vi "Display Print Dialog.vi"(8 "error in (no error)":errorcluster, 10 "WindowWrapper DLL Directory":path, 11 "Main VI":refnum<vi>) -> (0 "error out":errorcluster, 2 "PrinterName":string, 3 "Dialog result":i32(ring) items=["None", "OK", "Cancel", "Abort", "Retry", "Ignore", "Yes", "No"])   [LabVIEW 2013, in "Win32 Util.lvlib"]
doc: "Have to pass in the directory that WindowWrapper .NET DLL resides in otherwise get strange file not found errors."
uses:
  Win32 Util.lvlib
  System.Windows.Forms
  System.Drawing
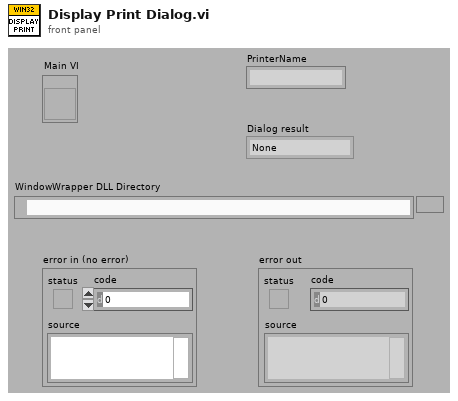
[diagram p1: front panel]
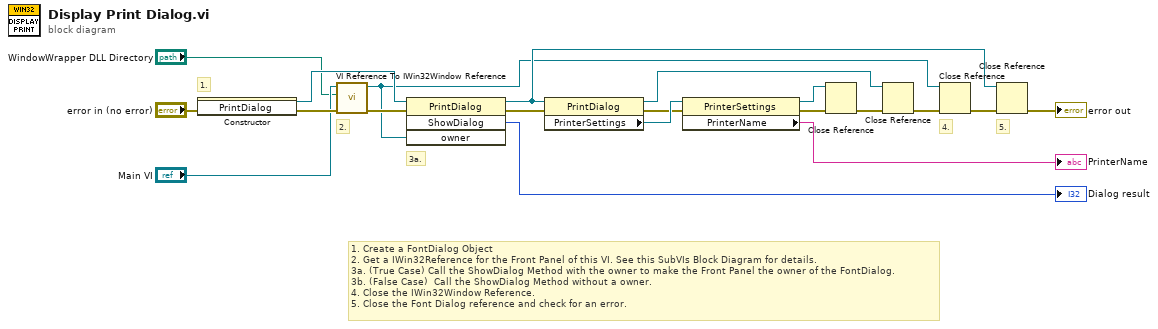
[diagram p0: block diagram]
diagram:
  # "4."
  # "3a."
  # "2."
  # "5."
  # "1. Create a FontDialog Object\n2. Get a IWin32Reference for the Front Panel of this VI. See this SubVIs Block Diagram for details. \n3a. (True Case) Call the ShowDialog Method with the owner to make the Front Panel the owner of the FontDialog.\n3b. (False Case)  Call the ShowDialog Method without a owner.\n4. Close the IWin32Window Reference.\n5. Close the Font Dialog reference and check for an error."
  # "1."
  n1 = constructor class="PrintDialog"(error in="error in (no error)") -> (reference out=w20:refnum<k24>, error out=w19:errorcluster)  [unwired: 2 in, 1 out]
  n2 = call "VI Reference To IWin32Window Reference.vi"("error in (no error)"=w19, "WindowWrapper DLL Directory"="WindowWrapper DLL Directory", "VI Reference"="Main VI") -> ("error out"=w15:errorcluster, "System.Windows.Forms.IWin32Window"=w14:refnum<k24>)  [unwired: 7 in]
  n3 = invoke class="PrintDialog" method="ShowDialog"(reference=w20, error in=w15, "owner"=w14) -> (reference out=w17:refnum<k24>, error out=w11:errorcluster, "ShowDialog"=→"Dialog result":i32)  [unwired: 1 in, 1 out]
  n4 = property class="PrintDialog"(reference=w17, error in=w11) -> (reference out=w6:refnum<k24>, error out=w10:errorcluster, "PrinterSettings"=w13:refnum<k24>)
  n5 = property class="PrinterSettings"(reference=w13, error in=w10) -> (reference out=w7:refnum<k24>, error out=w9:errorcluster, "PrinterName"=→"PrinterName":string)
  n6 = Close Reference(reference=w7, error in (no error)=w9) -> (error out=w8:errorcluster)
  n7 = Close Reference(reference=w6, error in (no error)=w8) -> (error out=w5:errorcluster)
  n8 = Close Reference(reference=w14, error in (no error)=w5) -> (error out=w18:errorcluster)
  n9 = Close Reference(reference=w17, error in (no error)=w18) -> (error out=→"error out":errorcluster)
